vi "Convert_data_to_string.vi"(0 "Data":T1, 5 "Wavelenght [nm]":dbl format="%#_13g", 7 "Min/Max Voltage [V]":dbl format="%#_13g", 9 "X Shift [V]":dbl format="%#_13g", 11 "Y Shift [V]":dbl format="%#_13g") -> (4 "spreadsheet string":string)   [LabVIEW 2021]
doc: "This VI enables to convert the measurements data to a string.\n\nInput:\n(1) Data: the data cluster.\nThis cluster contains the Threshold power [W], the number of seconds from the beginning and the measurement time stamp.\n\nOutput:\n(1) Spreadsheet string - the string which contains the measurement data"
uses:
  Data.ctl
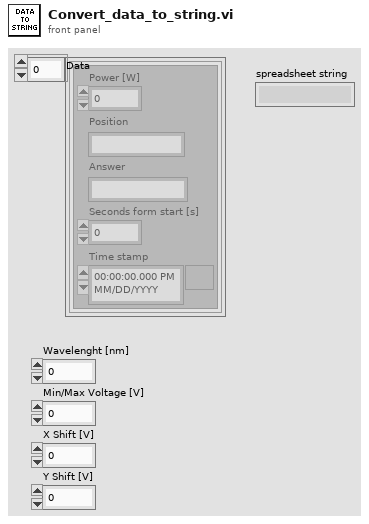
[diagram p1: front panel]
types:
  T1 = typedef "Data.ctl" = cluster{cluster{"Power [W]":dbl, "Position":string, "Answer":string, "Seconds form start [s]":dbl, "Time stamp":timestamp}}[]
  T2 = cluster{"Power [W]":dbl, "Position":string, "Answer":string, "Seconds form start [s]":dbl, "Time stamp":timestamp}
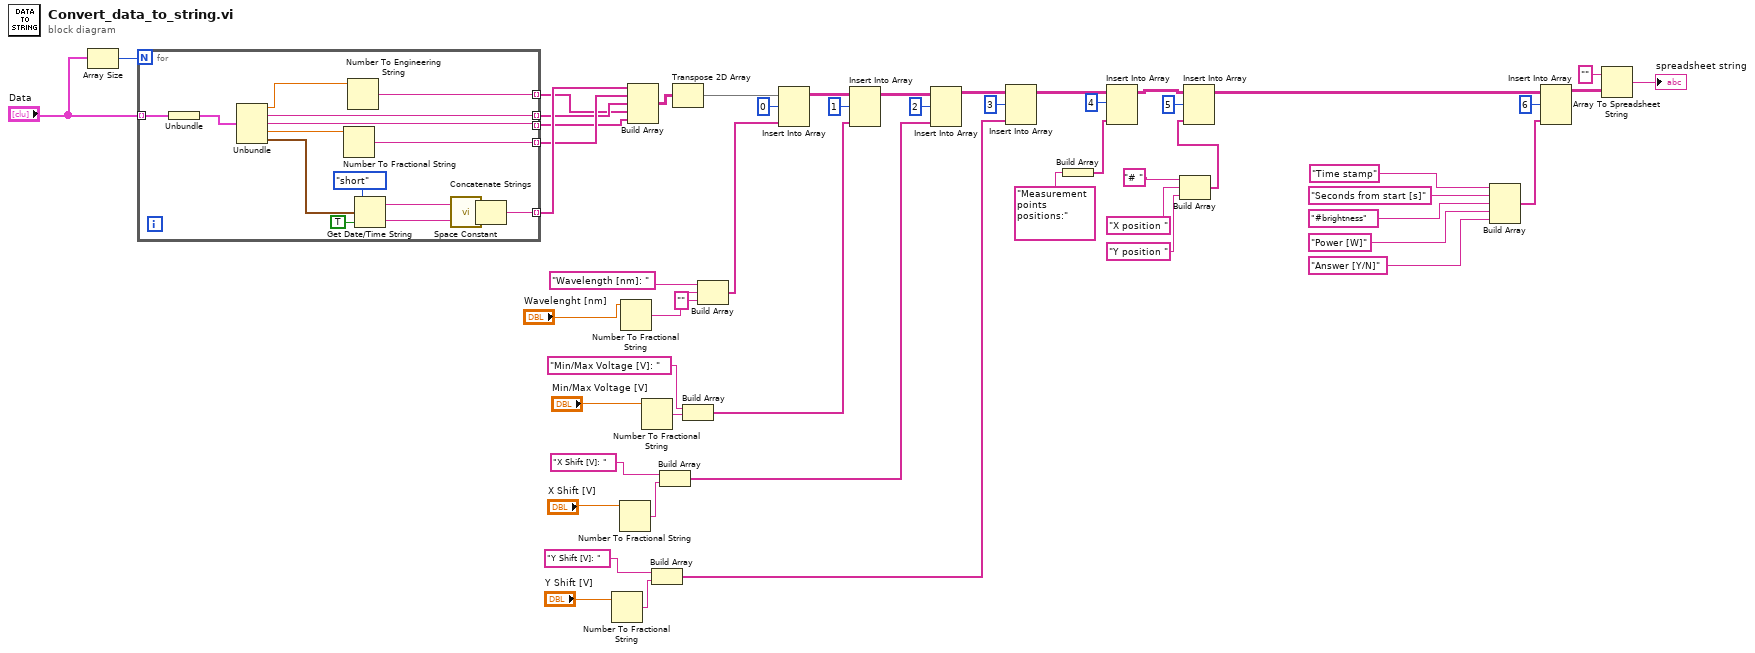
[diagram p0: block diagram]
diagram:
  n1 = Array Size(array="Data") -> (size(s)=w45:i32)
  n2 = for {
    N: w45 -> [_]
    tunnel: "Data" -> [w65] mode=indexing
    tunnel: [w59] -> w15 mode=indexing
    tunnel: [w60] -> w53 mode=indexing
    tunnel: [w61] -> w54 mode=indexing
    tunnel: [w58] -> w17 mode=indexing
    tunnel: [w55] -> w16 mode=indexing
    n3 = Unbundle(w65) -> (w69:T2)
    n4 = Unbundle(w69) -> ("Power [W]"=w66:dbl, "Position"=w58:string, "Answer"=w55:string, "Seconds form start [s]"=w56:dbl, "Time stamp"=w57:timestamp)
    n5 = Number To Fractional String(number=w56) -> (F-format string=w60:string)  [unwired: 3 in]
    n6 = Number To Engineering String(4:w66) -> (0:w59:string)  [unwired: 3 in]
    n7 = Get Date/Time String(date format (0)=enum16{"short", "long", "abbreviated"}."short", seconds (now)=w57, want seconds? (F)=TRUE) -> (date string=w64:string, time string=w62:string)
    n8 = call <vilib>:"Space Constant.vi"() -> ("String"=w63:string)
    n9 = Concatenate Strings(w64, w63, w62) -> (w61:string)
  }
  n10 = Number To Fractional String(number="Y Shift [V]") -> (F-format string=w21:string)  [unwired: 3 in]
  n11 = Number To Fractional String(number="X Shift [V]") -> (F-format string=w27:string)  [unwired: 3 in]
  n12 = Number To Fractional String(number="Wavelenght [nm]") -> (F-format string=w39:string)  [unwired: 3 in]
  n13 = Build Array(w54, w53, w17, w15, w16) -> (w50:string[][])
  n14 = Number To Fractional String(number="Min/Max Voltage [V]") -> (F-format string=w30:string)  [unwired: 3 in]
  n15 = Build Array("Y Shift [V]: " ("element"), w21) -> (w24:string[])
  n16 = Build Array("X Shift [V]: " ("element"), w27) -> (w26:string[])
  n17 = Transpose 2D Array(2D array=w50) -> (transposed array=w44:string[][])
  n18 = Build Array("Min/Max Voltage [V]: " ("element"), w30) -> (w31:string[])
  n19 = Build Array("Wavelength [nm]: ", w39, "" ("element")) -> (w42:string[])
  n20 = Insert Into Array(array=w44, index (row)=0, new element=w42) -> (w35:string[][])  [unwired: 1 in]
  n21 = Insert Into Array(array=w35, index (row)=1, new element=w31) -> (w34:string[][])  [unwired: 1 in]
  n22 = Insert Into Array(array=w34, index (row)=2, new element=w26) -> (w33:string[][])  [unwired: 1 in]
  n23 = Insert Into Array(array=w33, index (row)=3, new element=w24) -> (w14:string[][])  [unwired: 1 in]
  n24 = Build Array("Measurement points positions:" ("element")) -> (w8:string[])
  n25 = Insert Into Array(array=w14, index (row)=4, new element=w8) -> (w5:string[][])  [unwired: 1 in]
  n26 = Build Array("# " ("element"), "X position " ("element"), "Y position " ("element")) -> (w12:string[])
  n27 = Insert Into Array(array=w5, index (row)=5, new element=w12) -> (w2:string[][])  [unwired: 1 in]
  n28 = Build Array("Time stamp", "Seconds from start [s]", "#brightness", "Power [W]", "Answer [Y/N]" ("element")) -> (w48:string[])
  n29 = Insert Into Array(array=w2, index (row)=6, new element=w48) -> (w49:string[][])  [unwired: 1 in]
  n30 = Array To Spreadsheet String(array=w49, 3:"" ("format string")) -> (spreadsheet string=→"spreadsheet string":string)  [unwired: 1 in]
